vi "Actor Core.vi"(8 "error in":errorcluster, 11 "Nested in":refnum<class "Panel.lvclass">) -> (0 "error out":errorcluster, 3 "Actor out":refnum<class "Actor.lvclass">)   [LabVIEW 2021, in "Panel.lvlib" / "Panel.lvclass"]
doc: "(<B>Filename</B>: Actor Framework.lvlib:Actor.lvclass:Actor Core.vi)\n\nReceives messages to the actor, reacts to them, and initiates any error handling that may shut the actor down.\n\nDescendant classes may override this VI to append parallel tasks for the actor to complete while it handles messages. Overrides use the Call Parent Method node."
uses:
  Panel.lvclass
  C:/Program Files/National Instruments/LabVIEW 2021/vi.lib/ActorFramework/Actor/Actor.lvclass
  <vilib>/ActorFramework/Actor/Actor.lvclass
  Type Defs/Tester Rx Dataset.ctl
  Type Defs/Tester Tx Dataset.ctl
  Panel.lvclass/Panel.ctl
  <vilib>/ActorFramework/Actor/Actor.lvclass/Actor.ctl
  <vilib>/ActorFramework/Message Enqueuer/Message Enqueuer.lvclass/Message Enqueuer.ctl
  Panel Messages/Set Tester Rx Msg/Set Tester Rx Msg.lvclass/Set Tester Rx Msg.ctl
  Panel Messages/Set Tester Tx Msg/Set Tester Tx Msg.lvclass/Set Tester Tx Msg.ctl
  Panel Messages/Pause Resume OPC UA Msg/Pause Resume OPC UA Msg.lvclass/Pause Resume OPC UA Msg.ctl
  <vilib>/ActorFramework/Message Enqueuer/Init from Existing Queue.vi
  <vilib>/ActorFramework/Message Enqueuer/Enqueue.vi
  Panel Messages/Set Tester Rx Msg/Set Tester Rx Msg.lvclass
  C:/Program Files/National Instruments/LabVIEW 2021/vi.lib/ActorFramework/Message/Message.lvclass
  Panel Messages/Reinitalize Components Msg/Reinitalize Components Msg.lvclass
  Panel Messages/Set Tester Tx Msg/Set Tester Tx Msg.lvclass
  Panel Messages/Pause Resume OPC UA Msg/Pause Resume OPC UA Msg.lvclass
  <vilib>/ActorFramework/Stop Msg/Stop Msg.lvclass
  <vilib>/ActorFramework/Message Priority Queue/Priority Enqueue.vi
  Station/Station Actor/Station.lvclass
  <vilib>/ActorFramework/Message Enqueuer/Message Enqueuer.lvclass
panel:
  in  "Auto":bool
  in  "Reset":bool
  in  "Run":bool
  out "Tester Tx":T1
  in  "Tester Rx":T2={"Start"=FALSE, "NestStatus"=FALSE, "PalletID"=0, "BarcodeData"="P:10-000001R:04S:QMC2200001", "StepEcho"=0, "Cylinder_1"=FALSE, "Cylinder_2"=FALSE, "Cylinder_3"=FALSE, "Cylinder_4"=FALSE, "Cylinder_5"=FALSE, "ResultsAck"=FALSE, "Reset"=FALSE, "Stop"=FALSE, "FaultCode"=0}
  # "or reset"
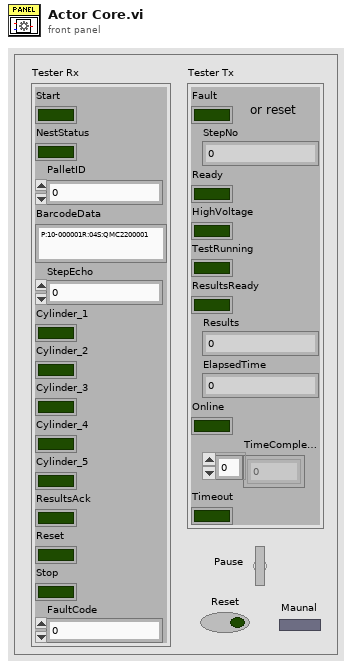
[diagram p1: front panel]
types:
  T1 = typedef "Panel.lvlib/Panel.lvclass/Tester Tx Dataset.ctl" = cluster{"Fault":bool, "StepNo":u32, "Ready":bool, "HighVoltage":bool, "TestRunning":bool, "ResultsReady":bool, "Results":u32, "ElapsedTime":u32, "Online":bool, "TimeCompleted":i32[], "Timeout":bool}
  T2 = typedef "Panel.lvlib/Panel.lvclass/Tester Rx Dataset.ctl" = cluster{"Start":bool, "NestStatus":bool, "PalletID":u32, "BarcodeData":string, "StepEcho":u32, "Cylinder_1":bool, "Cylinder_2":bool, "Cylinder_3":bool, "Cylinder_4":bool, "Cylinder_5":bool, "ResultsAck":bool, "Reset":bool, "Stop":bool, "FaultCode":u32}
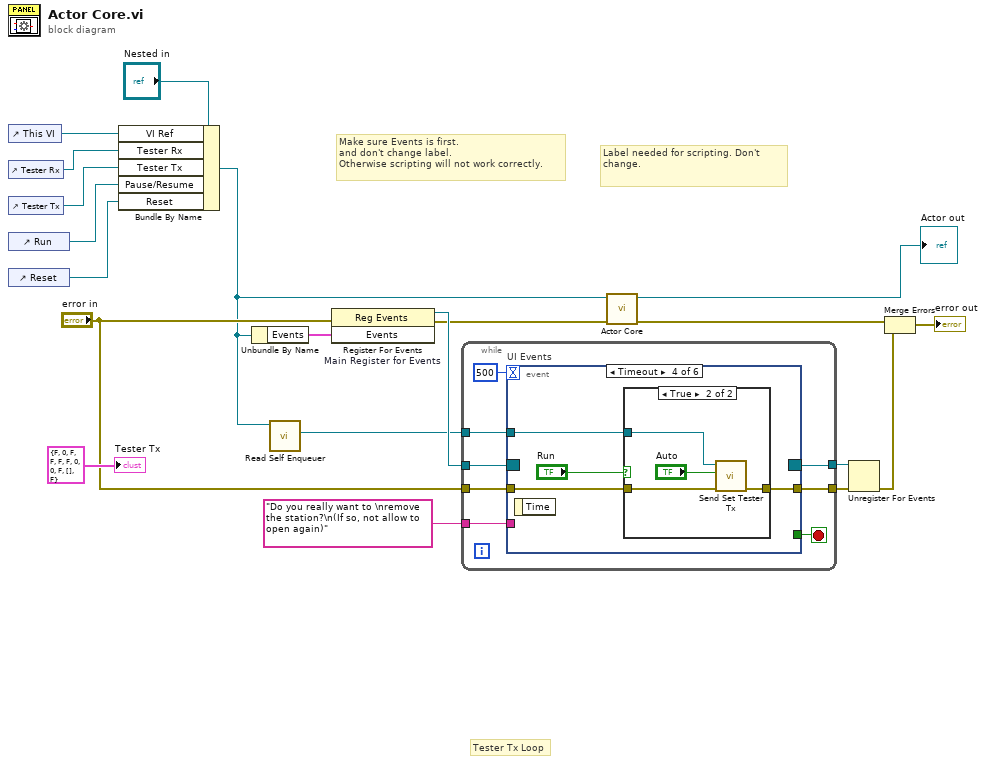
[diagram p0: block diagram]
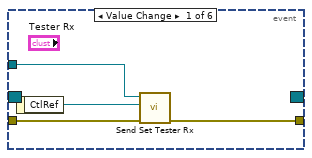
[diagram p2: hidden frame]
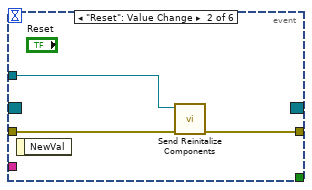
[diagram p3: hidden frame]
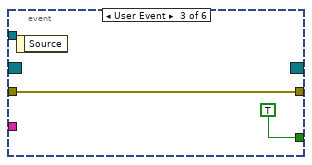
[diagram p4: hidden frame]
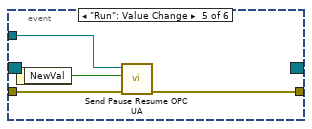
[diagram p6: hidden frame]
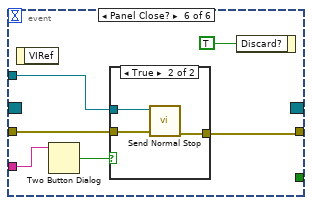
[diagram p7: hidden frame]
diagram:
  # "Tester Tx Loop"
  # "Label needed for scripting. Don't change."
  # "Make sure Events is first.\nand don't change label.\nOtherwise scripting will not work correctly."
  n1 = control-ref of="This VI"() -> (w15:refnum<vi>)
  n2 = control-ref of="Tester Rx"() -> (w13:refnum<vi>)
  n3 = control-ref of="Tester Tx"() -> (w12:refnum<vi>)
  n4 = control-ref of="Run"() -> (w7:refnum<vi>)
  n5 = control-ref of="Reset"() -> (w2:refnum<vi>)
  n6 = Bundle By Name(cluster="Nested in", "VI Ref"=w15, "Tester Rx"=w13, "Tester Tx"=w12, "Pause/Resume"=w7, "Reset"=w2) -> (w1:refnum<class "Panel.lvclass">)
  n7 = Unbundle By Name(w1) -> ("Events"=w18:cluster{"Stop":refnum<user-event>})
  n8 = call <vilib>:"Read Self Enqueuer.vi"("Actor"=w1) -> ("Self Enqueuer"=w6:refnum<class "Message Enqueuer.lvclass">)  [unwired: 10 in]
  n9 = register-events "Main Register for Events"(error in="error in", w18) -> (reference out=w19:refnum<event-registration>, error out=w4:errorcluster)  [unwired: 1 in]
  n10 = while {
    tunnel: w19 -> [w28]
    tunnel: [w26] -> w17
    tunnel: w6 -> [w25]
    tunnel: "error in" -> [w24]
    tunnel: [w23] -> w9
    tunnel: "Do you really want to \nremove the station?\n(If so, not allow to open again)" ("message") -> [w21]
    stop <- w27 stop-if-true
    n11 = event "UI Events" shown="[3] Timeout" {
      selector: w28 -> [_ _ _ _ _ _]
      dyn-events: [_ _ _ _ _ _] -> w26
      timeout: 500 -> [_ _ _ _ _ _]
      tunnel: [_ _ TRUE _ _ _] -> w27
      tunnel: w25 -> [w32 w33 _ w39 w50 w55]
      tunnel: w24 -> [w30 w35 w36 w41 w49 w54]
      tunnel: [w29 w34 w36 w40 w48 w53] -> w23
      tunnel: w21 -> [_ _ _ _ _ w51]
      event Value Change {
        n12 = event-data() -> ("CtlRef"=w31:refnum<vi>)  [unwired: 1 in]
        n13 = call "Send Set Tester Rx.vi"("error in (no error)"=w30, "ctl ref"=w31, "Message Enqueuer"=w32) -> ("error out"=w29:errorcluster)  [unwired: 7 in, 1 out]
      }
      event "Reset": Value Change {
        n14 = event-data() -> ()  [unwired: 1 in, 1 out]
        n15 = call "Send Reinitalize Components.vi"("error in (no error)"=w35, "Message Enqueuer"=w33) -> ("error out"=w34:errorcluster)  [unwired: 8 in, 1 out]
      }
      event User Event {
        n16 = event-data() -> ()  [unwired: 1 in, 1 out]
      }
      event Timeout {
        n17 = event-data() -> ()  [unwired: 1 in, 1 out]
        n18 = case shown="True" "Run" {
          tunnel: w41 -> [w42 w46]
          tunnel: [w42 w45] -> w40
          tunnel: w39 -> [_ w44]
          frame False {
          }
          frame True {
            n19 = call "Send Set Tester Tx.vi"("error in (no error)"=w46, "Auto/Manual"="Auto", "Message Enqueuer"=w44) -> ("error out"=w45:errorcluster)  [unwired: 7 in, 1 out]
          }
        }
      }
      event "Run": Value Change {
        n20 = event-data() -> ("NewVal"=w47:bool)  [unwired: 1 in]
        n21 = call "Send Pause Resume OPC UA.vi"("error in (no error)"=w49, "Pause/Resume"=w47, "Message Enqueuer"=w50) -> ("error out"=w48:errorcluster)  [unwired: 7 in, 1 out]
      }
      event Panel Close? {
        n22 = event-data() -> ()  [unwired: 1 in, 1 out]
        n23 = Two Button Dialog(message=w51) -> (T button?=w52:bool)  [unwired: 2 in]
        n24 = case shown="True" w52 {
          tunnel: w55 -> [_ w60]
          tunnel: w54 -> [w57 w59]
          tunnel: [w57 w58] -> w53
          frame False {
          }
          frame True {
            n25 = call <vilib>:"Send Normal Stop.vi"("error in (no error)"=w59, "Message Enqueuer"=w60) -> ("error out"=w58:errorcluster)  [unwired: 9 in]
          }
        }
        n26 = event-data("Discard?"=TRUE) -> ()  [unwired: 1 in, 1 out]
      }
    }
  }
  n27 = call-parent "Actor Core.vi"("error in"=w4, "Station in"=w1) -> ("error out"=w11:errorcluster, "Actor out"=→"Actor out":refnum<class "Actor.lvclass">)  [unwired: 8 in]
  n28 = Unregister For Events(event registration refnum=w17, error in=w9) -> (error out=w8:errorcluster)
  n29 = Merge Errors(w11, w8) -> (→"error out":errorcluster)
  "Tester Tx" <- T1 {"Fault"=FALSE, "StepNo"=0, "Ready"=FALSE, "HighVoltage"=FALSE, "TestRunning"=FALSE, "ResultsReady"=FALSE, "Results"=0, "ElapsedTime"=0, "Online"=FALSE, "TimeCompleted"=[], "Timeout"=FALSE} ("Tester Tx")
